vi "Degaussing FM with NI USB-6211.vi"() -> ()   [LabVIEW 2011]
doc: "I. Description:\nThis example demonstrates how to continuously output a waveform using an internal sample clock. The automatic regeneration of data has been disabled, so new data has to be provided throughout the duration of the continuous Analog Output operation. This allows the generation of any arbitrary frequency as this VI computes new data for each iteration of the loop, maintaining phase continuity of the signal.\n\nII. Instructions for Running:\n1. Select the Physical Channel to correspond to where your signal is output on the DAQ device.\n2. Enter the Minimum and Maximum Voltage range.\n3. Specify the desired Sample Clock Rate of the output Waveform. Higher sample clock rates will produce a smoother waveform.\n4. Manually specify the Analog Output buffer size, in number of samples. A larger buffer would help non-regenerative operations avoid errors due to occasional high CPU load. \nNote: \nThe Analog Output buffer has to be at least as big as the amount of data being written to the board per iteration. The recommended buffer size would be at least twice the amount of data being written to the board per iteration.\n5. Enter the Waveform Information. See the documentation of the Basic Function Generator SubVI for information on each parameter.\n\nIII. Block Diagram Steps:\n1. Create an Analog Output Voltage channel.\n2. Configure the task to prohibit the automatic regeneration of data.\n3. Call the DAQmx (Sample Clock) VI to set the sample clock rate. Additionally, set the sample mode to Continuous.\n4. Read the actual sample clock rate (eventually coerced depending on the hardware used). \n5. Compute the desired waveform, using the buffer size and the actual update rate. This VI keeps track of the phase of the waveform to ensure that the generated signal is continuous.\n6. Write the waveform to the output buffer. \n7a. Call the Start VI. This is only needed when the loop is executed for the first time.\n7b. Do nothing.\n8. Loop continuously until user presses the Stop button. Every iteration computes and writes a new waveform to the buffer.\n9. Call the Clear Task VI to clear the Task.\n10. Use the popup dialog box to display an error or warning if any.\n\nIV. I/O Connections Overview:\nMake sure your signal output terminal matches the Physical Channel I/O Control. For further connection information, refer to your hardware reference manual."
uses:
  <vilib>/Utility/error.llb/DialogType.ctl
  <vilib>/DAQmx/write.llb/DAQmx Write (Analog Wfm 1Chan NSamp).vi
  <vilib>/DAQmx/create/channels.llb/DAQmx Create Channel (AO-Voltage-Basic).vi
  <vilib>/DAQmx/configure/timing.llb/DAQmx Timing (Sample Clock).vi
  <vilib>/DAQmx/miscellaneous.llb/DAQmx Fill In Error Info.vi
  Programme/National Instruments/LabVIEW 2011/resource/objmgr/daqmx.rc
  <vilib>/measure/NI_MABase.lvlib
  WinAccCouchDB/Debug/WinAccCouchDB.dll
panel:
  out "value":dbl
  in  "Stop":bool
  out "Abort 2":i32
  out "Abort":dbl
  out "Offset":dbl
  in  "Amplitude":dbl=10.0 format="%.2f"
  in  "Phase":dbl format="%3_3g"
  in  "End f":dbl=10.0 caption="End  f" format="%.2f"
  in  "Waveform Type 2":T1(ring) caption="Waveform Type"
  in  "Start f":dbl=10.0 caption="Start  f" format="%.2f"
  in  "c":dbl=1.0 caption="Keep, s"
  in  "a":dbl=100.0 caption="Increase, s"
  in  "b":dbl=1000.0 caption="Decrease, s"
  out "Envelope Output":waveform(dbl)(graph)={"t0"=timestamp(1201.1000000000001 s since 1904-01-01), "dt"=5e-05, "Y"=array[2000 elements]}
  in  "Size (Samples)":u32=2000 caption="Samples"
  out "Actual":dbl=20000.0 format="%.2f"
  in  "Sample Clock Rate":dbl=20000.0 format="%0.2f"
  out "Waveform Graph":waveform(dbl)(graph)={"t0"=timestamp(1201.1000000000001 s since 1904-01-01), "dt"=5e-05, "Y"=array[2000 elements]} caption="Generated Waveform"
  in  "Physical Channels":tag="Dev3/ao0"
  in  "Minimum Value":dbl=-10.0 format="%0.2f"
  in  "Maximum Value":dbl=10.0 format="%0.2f"
  in  "stop":bool
  # "Degaussing waveform generator with NI USB-6211 analog output"
  # "Channel Parameters"
  # "Timing Parameters"
  # "Envelope Parameters"
  # "Control via CouchApp"
  # "Buffer Parameters"
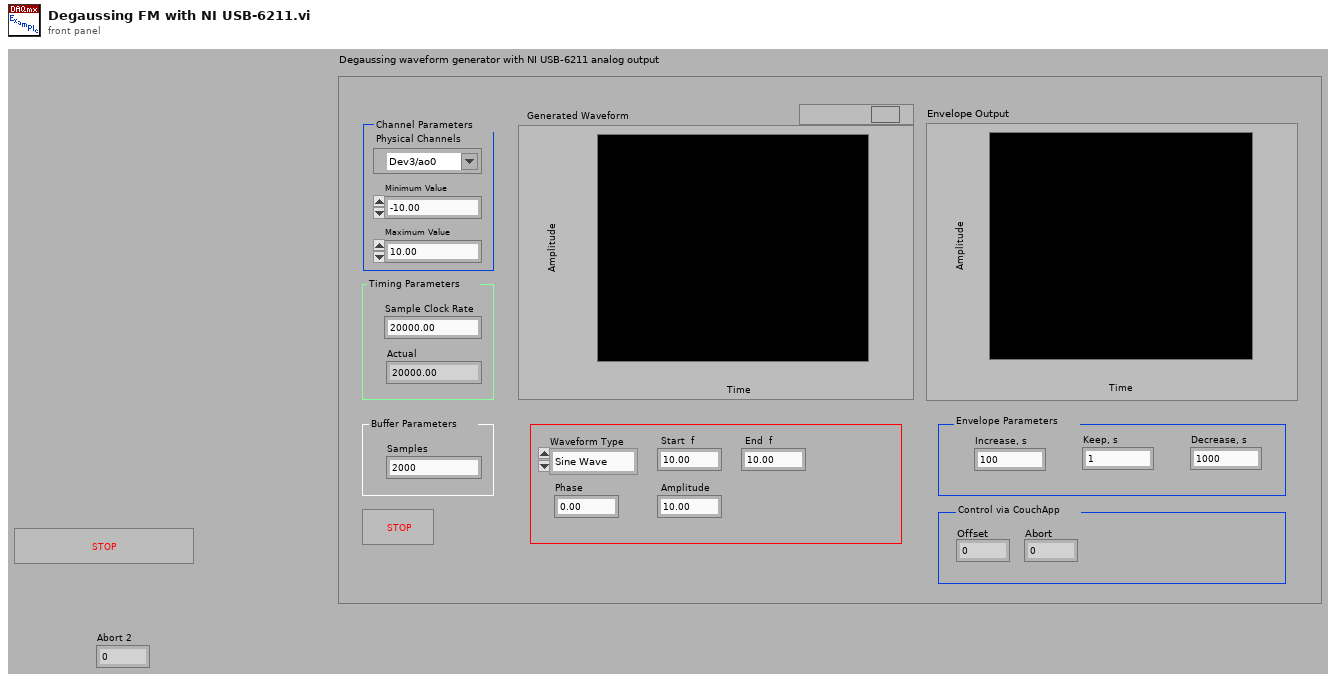
[diagram p1: front panel]
types:
  T1 = enum16{"Sine Wave", "Triangle Wave", "Square Wave", "Sawtooth Wave"}
  T2 = typedef "DialogType.ctl" = u16
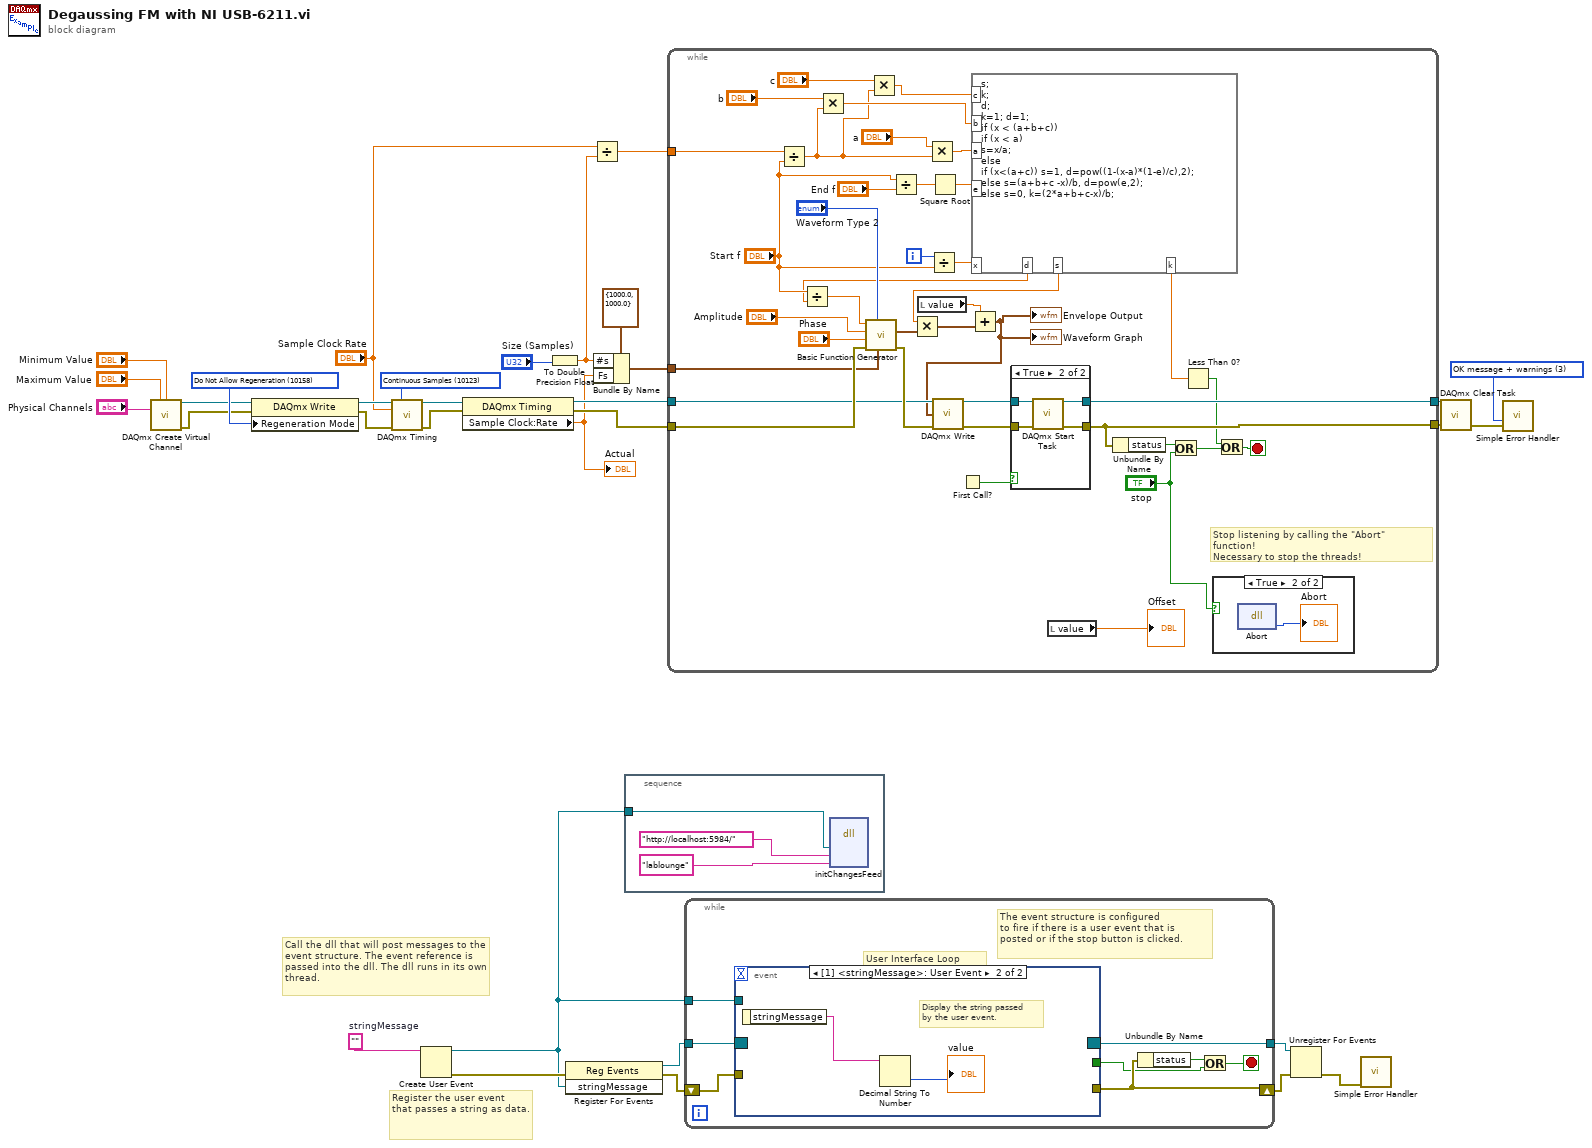
[diagram p0: block diagram]
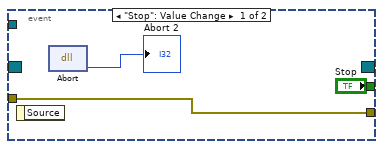
[diagram p2: hidden frame]
diagram:
  w1 = ""  # stringMessage
  w20 = 10158 items=["Allow Regeneration"=10097, "Do Not Allow Regeneration"=10158] ("RegenMode")
  w27 = T2 3 items=["no dialog", "OK message", "continue or stop message", "OK message + warnings", "continue/stop + warnings"] ("type of dialog (OK msg:1)")
  w31 = 10123 items=["Finite Samples"=10178, "Continuous Samples"=10123] ("sample mode")
  # "Call the dll that will post messages to the event structure. The event reference is passed into the dll. The dll runs in its own thread."
  # "Register the user event \nthat passes a string as data."
  n1 = call-poly <vilib>:"DAQmx Create Virtual Channel.vi"("maximum value"="Maximum Value", "minimum value"="Minimum Value", "physical channels"="Physical Channels") -> ("task out"=w19:refnum<k21>, "error out"=w18:errorcluster)  [unwired: 11 in]
  n2 = property class="DAQmx Write"(reference=w19, error in=w18, "Regeneration Mode"=w20) -> (reference out=w14:refnum<k21>, error out=w13:errorcluster)
  n3 = call-poly <vilib>:"DAQmx Timing.vi"("task/channels in"=w14, "sample mode"=w31, "rate"="Sample Clock Rate", "error in"=w13) -> ("task out"=w24:refnum<k21>, "error out"=w23:errorcluster)  [unwired: 10 in]
  n4 = Create User Event(user event datatype=w1) -> (user event=w2:refnum<user-event>, error out=w3:errorcluster)  [unwired: 1 in]
  n5 = property class="DAQmx Timing"(reference=w24, error in=w23) -> (reference out=w17:refnum<k21>, error out=w16:errorcluster, "Sample Clock:Rate"=w12:dbl)
  "Actual" <- w12
  n6 = To Double Precision Float(number="Size (Samples)") -> (double precision float=w11:dbl)
  n7 = register-events(error in=w3, w2) -> (reference out=w6:refnum<event-registration>, error out=w4:errorcluster)  [unwired: 1 in]
  n8 = Divide(x="Sample Clock Rate", y=w11) -> (x/y=w9:dbl)
  n9 = Bundle By Name(cluster=cluster{"Fs":dbl, "#s":dbl} {"Fs"=1000.0, "#s"=1000.0} ("sampling info"), "#s"=w11, "Fs"=w12) -> (w21:cluster{"Fs":dbl, "#s":dbl})
  n10 = stacked-sequence {
    tunnel: w2 -> [w33]
    frame #0 {
      n11 = dll-call lib="C:/projects/WinAccCouchDB/Debug/WinAccCouchDB.dll" fn="initChangesFeed"("UserEventRef"=w33, "server"="http://localhost:5984/", "database"="lablounge") -> ()  [unwired: 7 in, 2 out]
    }
  }
  n12 = while {
    tunnel: w17 -> [w71]
    tunnel: [w67] -> w26
    tunnel: w16 -> [w74]
    tunnel: [w68] -> w25
    tunnel: w21 -> [w72]
    tunnel: w9 -> [w62]
    i -> [w64]
    stop <- w53 stop-if-true
    # "Stop listening by calling the \"Abort\" function!\nNecessary to stop the threads!"
    n13 = Divide(x=w62, y="Start f") -> (x/y=w50:dbl)
    n14 = Multiply(x="b", y=w50) -> (x*y=w60:dbl)
    n15 = Multiply(x="c", y=w50) -> (x*y=w49:dbl)
    n16 = Divide(x="Start f", y="End f") -> (x/y=w44:dbl)
    n17 = local read "value"() -> (w38:dbl)
    n18 = Multiply(x="a", y=w50) -> (x*y=w61:dbl)
    n19 = Divide(x=w64, y="Start f") -> (x/y=w63:dbl)
    n20 = Square Root(x=w44) -> (sqrt(x)=w43:dbl)
    n21 = First Call?() -> (First Call?: T/F=w66:bool)
    n22 = formula code="s;\nk; \nd;\nk=1; d=1;\nif (x < (a+b+c))\nif (x < a) \ns=x/a; \nelse \nif (x<(a+c)) s=1, d=pow((1-(x-a)*(1-e)/c),2); \nelse s=(a+b+c -x)/b, d=pow(e,2);\nelse s=0, k=(2*a+b+c-x)/b;"("a"=w61, "x"=w63, "b"=w60, "c"=w49, "e"=w43) -> ("s"=w52:dbl, "k"=w58:dbl, "d"=w40:dbl)
    n23 = Divide(x="Start f", y=w40) -> (x/y=w41:dbl)
    n24 = call <vilib>:"Basic Function Generator.vi"("sampling info"=w72, "signal type"="Waveform Type 2", "error in (no error)"=w74, "phase"="Phase", "amplitude"="Amplitude", "frequency"=w41) -> ("error out"=w73:errorcluster, "signal out"=w65:waveform(dbl))  [unwired: 3 in, 1 out]
    n25 = Multiply(x=w52, y=w65) -> (x*y=w59:waveform(dbl))
    n26 = Add(x=w38, y=w59) -> (x+y=w39:waveform(dbl))
    "Waveform Graph" <- w39
    "Envelope Output" <- w39
    n27 = call-poly <vilib>:"DAQmx Write.vi"("task/channels in"=w71, "data"=w39, "error in"=w73) -> ("task out"=w70:refnum<k21>, "error out"=w69:errorcluster)  [unwired: 10 in, 1 out]
    n28 = case shown="True" w66 {
      tunnel: w70 -> [w78 w82]
      tunnel: w69 -> [w77 w81]
      tunnel: [w77 w80] -> w68
      tunnel: [w78 w79] -> w67
      frame False {
        # "7b."
      }
      frame True {
        n29 = call <vilib>:"DAQmx Start Task.vi"("task/channels in"=w82, "error in"=w81) -> ("task out"=w79:refnum<k21>, "error out"=w80:errorcluster)  [unwired: 12 in]
      }
    }
    n30 = local read "value"() -> (→"Offset":dbl)
    n31 = Unbundle By Name(w68) -> ("status"=w75:bool)
    n32 = Or(x=w75, y="stop") -> (x .or. y?=w54:bool)
    n33 = Less Than 0?(x=w58) -> (x < 0?=w55:bool)
    n34 = case shown="True" "stop" {
      frame False {
      }
      frame True {
        n35 = dll-call lib="C:/projects/WinAccCouchDB/Debug/WinAccCouchDB.dll" fn="Abort"() -> ("return type"=→"Abort":i32)  [unwired: 3 in, 2 out]
      }
    }
    n36 = Or(x=w55, y=w54) -> (x .or. y?=w53:bool)
  }
  n37 = while {
    tunnel: w6 -> [w90]
    shift-right: [w88] -> w7
    shift-left: w4 -> [w89]
    tunnel: [w87] -> w5
    tunnel: w2 -> [w83]
    stop <- w85 stop-if-true
    # "The event structure is configured\nto fire if there is a user event that is\nposted or if the stop button is clicked."
    # "User Interface Loop"
    n38 = event shown="[1] <stringMessage>: User Event" {
      selector: w90 -> [_ _]
      dyn-events: [_ _] -> w87
      timeout: _ -> [_ _]
      tunnel: ["Stop" _] -> w84
      tunnel: w89 -> [w92 _]
      tunnel: [w92 _] -> w88
      tunnel: w83 -> [_ _]
      event "Stop": Value Change {
        n39 = event-data() -> ()  [unwired: 1 in, 1 out]
        n40 = dll-call lib="C:/projects/WinAccCouchDB/Debug/WinAccCouchDB.dll" fn="Abort"() -> ("return type"=→"Abort 2":i32)  [unwired: 3 in, 2 out]
      }
      event User Event {
        # "Display the string passed\nby the user event."
        n41 = event-data() -> ("stringMessage"=w95:string)  [unwired: 1 in]
        n42 = Decimal String To Number(string=w95) -> (number=→"value":i32)  [unwired: 2 in, 1 out]
      }
    }
    n43 = Unbundle By Name(w88) -> ("status"=w86:bool)
    n44 = Or(x=w86, y=w84) -> (x .or. y?=w85:bool)
  }
  n45 = Unregister For Events(event registration refnum=w5, error in=w7) -> (error out=w8:errorcluster)
  n46 = call <vilib>:"Simple Error Handler.vi"("error in (no error)"=w8) -> ()  [unwired: 4 in, 5 out]
  n47 = call <vilib>:"DAQmx Clear Task.vi"("task in"=w26, "error in"=w25) -> ("error out"=w32:errorcluster)  [unwired: 13 in]
  n48 = call <vilib>:"Simple Error Handler.vi"("type of dialog (OK msg:1)"=w27, "error in (no error)"=w32) -> ()  [unwired: 3 in, 5 out]
